vi "Vision Processing (1).vi"(4 "View Processed Image":bool, 5 "Image Size":i32, 6 "Score Limits":T5={"Rect Coverage"=60.0, "X Edge Strength"=40.0, "Y Edge Strength"=60.0, "Center"=75.0, "Outer"=75.0}, 7 "Camera Type":enum16{"206", "1011"}(ring)=enum."1011", 8 "Area Size Limit %":dbl=0.5, 9 "Particle Count Limit":i32=8, 10 "Image Filter Values":T2={"Hue"=89, "Saturation"=255, "Luminance"=255, "Margins"={"Hue"=80, "Val"=0, "Sat"=0}} {"Margins"."Sat" scale=0.0..80.0; "Margins"."Val" scale=0.0..80.0; "Margins"."Hue" scale=0.0..80.0; "Hue" scale=0.0..255.0}, 11 "Image In":T4) -> (1 "Image Filter Ranges":T1, 2 "Processed Image":T4(plugin-control), 3 "Target Info":T6(array[cluster]))   [LabVIEW 2013]
uses:
  <vilib>/vision/Image Controls.llb/IMAQ Image.ctl
  <vilib>/vision/NI_Vision_Development_Module.lvlib
panel:
  in  "Image Filter":T3
  in  "Processing":enum32{"Color", "Monochrome"}(tab)
  in  "Range":cluster{"Lower value":sgl, "Upper value":sgl}={"Lower value"=150.0, "Upper value"=255.0} {"Lower value" scale=0.0..255.0; "Upper value" scale=0.0..255.0}
  in  "View":bool
  out "Original Image":T4(plugin-control)
  # "<--- Disabled"
  # "Lower/Upper"
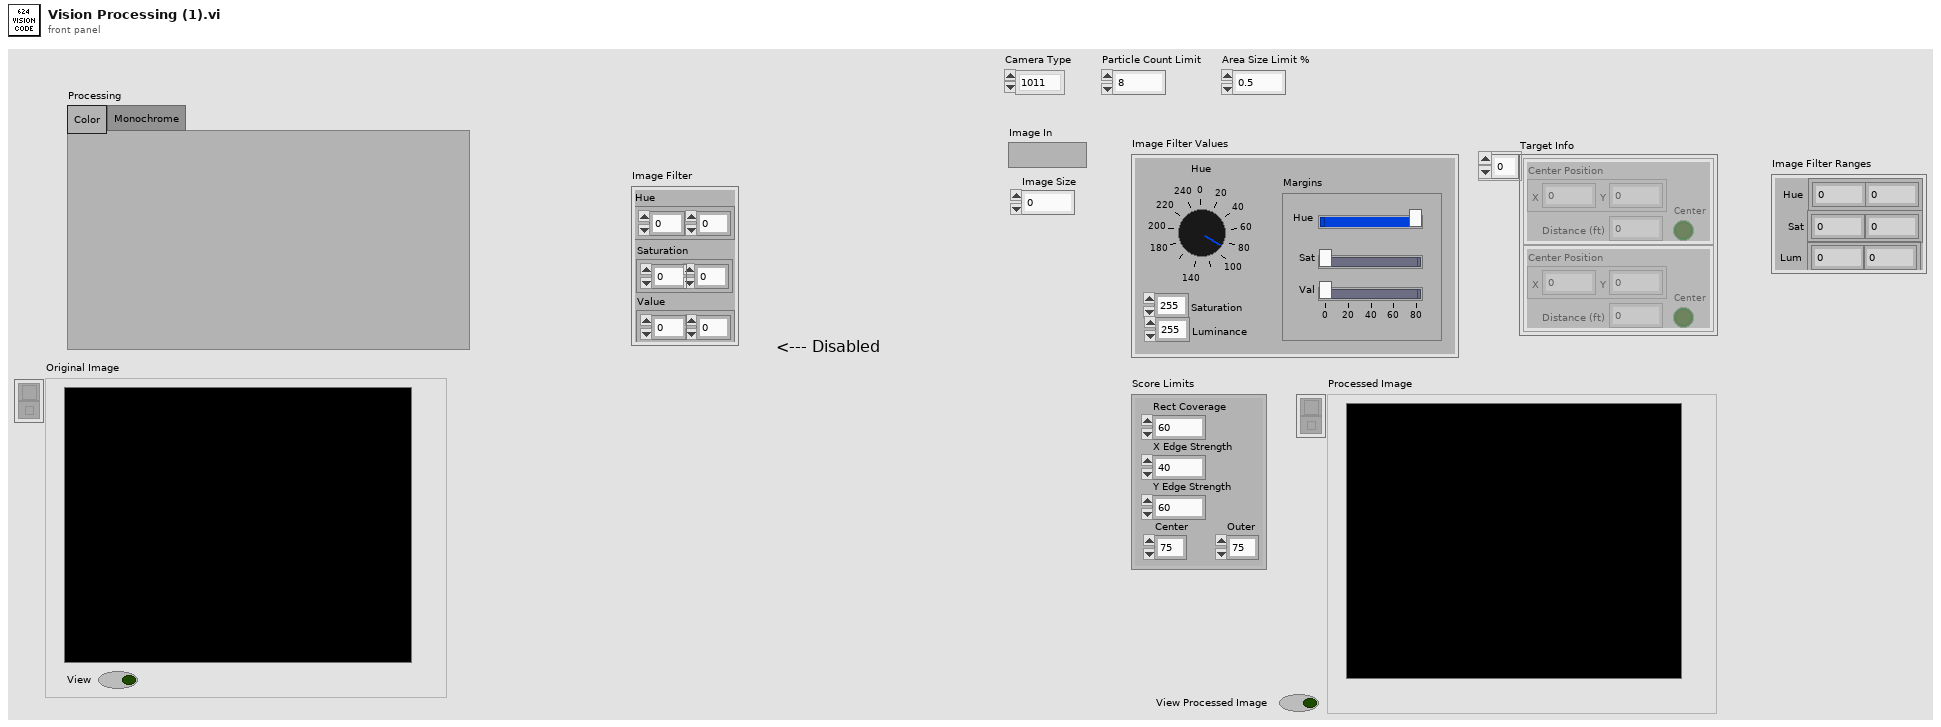
[diagram p1: front panel]
types:
  T1 = cluster{"Hue":cluster{i32, i32}, "Sat":cluster{i32, i32}, "Lum":cluster{i32, i32}}
  T2 = cluster{"Hue":i32, "Saturation":i32, "Luminance":i32, "Margins":cluster{"Hue":i32, "Val":i32, "Sat":i32}}
  T3 = cluster{"Hue":cluster{i32, i32}, "Saturation":cluster{i32, i32}, "Value":cluster{i32, i32}}
  T4 = typedef "IMAQ Image.ctl" = refnum<image>
  T5 = cluster{"Rect Coverage":dbl, "X Edge Strength":dbl, "Y Edge Strength":dbl, "Center":dbl, "Outer":dbl}
  T6 = cluster{"Center Position":cluster{"X":dbl, "Y":dbl}, "Distance (ft)":dbl, "Center":bool}[]
  T7 = cluster{"Position":cluster{"X":dbl, "Y":dbl}, "Distance (ft)":dbl, "Center":bool}[]
  T8 = typedef "Image Type" = u32
  T9 = cluster{cluster{"Left":dbl, "Top":dbl, "Right":dbl, "Bottom":dbl}, "Scores":dbl[], cluster{"Long":dbl, "Short":dbl}}[]
  T10 = cluster{"Target Center (-1 to 1)":cluster{"X":dbl, "Y":dbl}, "Distance (ft)":dbl, "Center Target":bool}
  T11 = cluster{"Target Center (-1 to 1)":cluster{"X":dbl, "Y":dbl}, "Distance (ft)":dbl, "Center Target":bool}[]
  T12 = cluster{"Left":dbl, "Top":dbl, "Right":dbl, "Bottom":dbl}
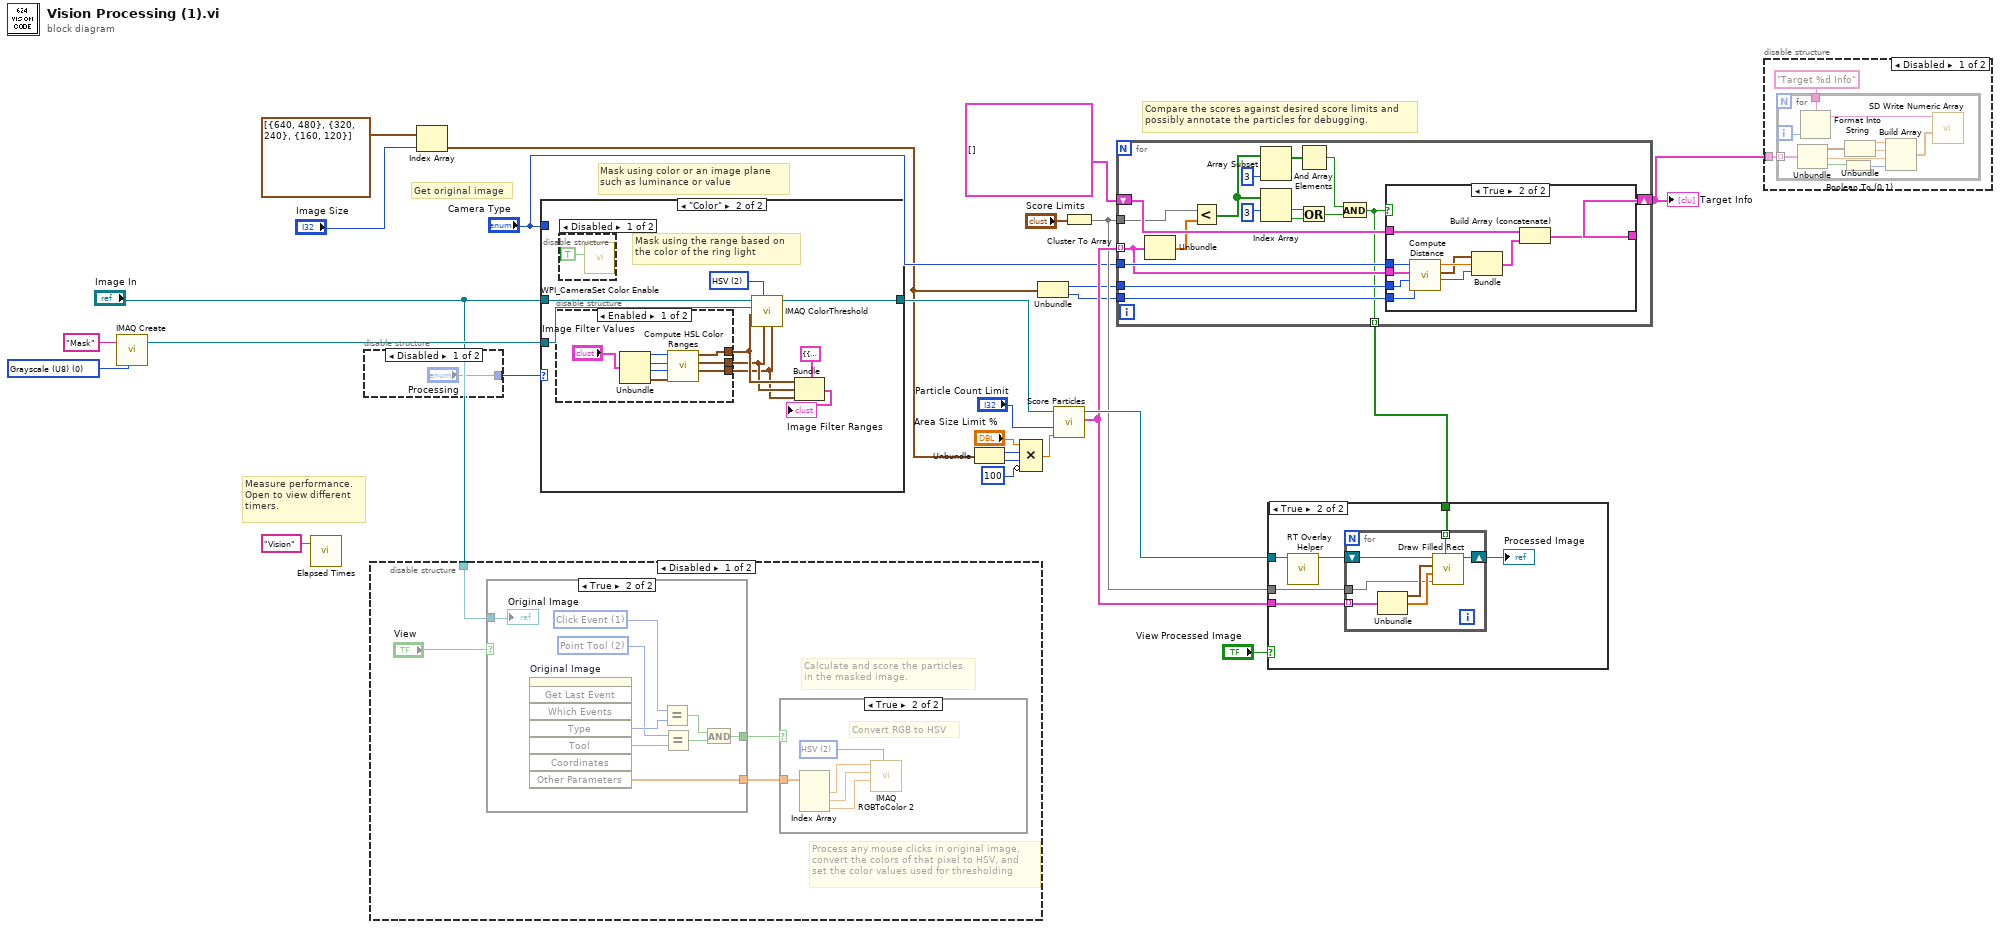
[diagram p0: block diagram]
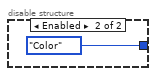
[diagram p8: hidden frame]
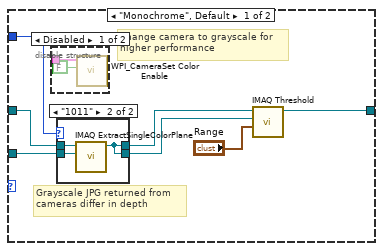
[diagram p9: hidden frame]
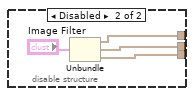
[diagram p12: hidden frame]
diagram:
  w27 = T8 0 items=["Grayscale (U8)", "Grayscale (I16)", "Grayscale (SGL)", "Complex (CSG)", "RGB (U32)", "HSL (U32)", "RGB (U64)", "Grayscale (U16)"] ("Image Type")
  # "Compare the scores against desired score limits and\npossibly annotate the particles for debugging."
  # "Mask using color or an image plane\nsuch as luminance or value"
  # "Get original image"
  # "Measure performance.\nOpen to view different\ntimers."
  n1 = call "IMAQ Create"("Image Name"="Mask", "Image Type"=w27) -> ("New Image"=w25:T4)  [unwired: 2 in, 2 out]
  n2 = call "Elapsed Times.vi"("Call Name"="Vision") -> ()  [unwired: 2 in, 1 out]
  n3 = disable-structure shown="Disabled" {
    disable-tunnel: ["Processing" enum32{"Color", "Monochrome"}."Color" ("Processing 2")] -> w22
    frame Disabled {
    }
    frame Enabled {
    }
  }
  n4 = disable-structure shown="Disabled" {
    disable-tunnel: "Image In" -> [w30 _]
    frame Disabled {
      # "Process any mouse clicks in original image,\nconvert the colors of that pixel to HSV, and\nset the color values used for thresholding"
      # "Calculate and score the particles\nin the masked image."
      n5 = case shown="True" "View" {
        tunnel: w30 -> [_ w47]
        tunnel: [_ w42] -> w32
        tunnel: [_ w39] -> w31
        frame False {
        }
        frame True {
          w40 = 2 items=["None", "Selection Tool", "Point Tool", "Line Tool", "Rectangle Tool", "Oval Tool", "Polygon Tool", "ClosedFreehandTool", "Annulus Tool", "Rotated Rectangle Tool", "Zoom Tool", "Pan Tool", "Polyline Tool", "Freehand Tool"] ("Tool")
          w41 = 1 items=["No Event"=0, "Click Event"=1, "Draw Event"=2, "Size Event"=4, "Scroll Event"=5, "Double Click Event"=8] ("Type")
          n6 = invoke on="Original Image" class="ImageControl" method="Get Last Event"() -> ("Type"=w43:i32, "Tool"=w46:i32, "Other Parameters"=w39:sgl[])  [unwired: 8 in, 5 out]
          n7 = Equal?(x=w41, y=w43) -> (x = y?=w44:bool)
          n8 = Equal?(x=w40, y=w46) -> (x = y?=w45:bool)
          n9 = And(x=w44, y=w45) -> (x .and. y?=w42:bool)
          "Original Image" <- w47
        }
      }
      n10 = case shown="True" w32 {
        tunnel: w31 -> [_ w38]
        frame False {
        }
        frame True {
          w37 = u16 2 items=["RGB", "HSL", "HSV", "HSI", "CIE L*a*b*", "CIE XYZ"] ("Color Mode")
          # "Convert RGB to HSV"
          n11 = Index Array(array=w38) -> (element #1=w36:sgl, element #2=w35:sgl, element #3=w34:sgl)  [unwired: 3 in]
          n12 = call "IMAQ RGBToColor 2"("Color Mode"=w37, "Blue value"=w34, "Green value"=w35, "Red value"=w36) -> ()  [unwired: 4 in, 4 out]
        }
      }
    }
    frame Enabled {
    }
  }
  n13 = Index Array(array=cluster{i32, i32}[] [{640, 480}, {320, 240}, {160, 120}], index="Image Size") -> (element=w15:cluster{i32, i32})
  n14 = case shown="\"Color\"" w22 {
    tunnel: "Image In" -> [w52 w70]
    tunnel: [w53 w69] -> w18
    tunnel: w25 -> [w51 w67]
    tunnel: "Camera Type" -> [w50 _]
    frame "Monochrome", Default {
      # "Grayscale JPG returned from\ncameras differ in depth"
      # "Change camera to grayscale for\nhigher performance"
      n15 = disable-structure shown="Disabled" {
        disable-tunnel: _ -> [w55 _]
        frame Disabled {
          n16 = call <vilib>:"WPI_CameraSet Color Enable.vi"("Color Enabled"=FALSE, "CameraDevRef"=w55) -> ()  [unwired: 8 in, 2 out]
        }
        frame Enabled {
        }
      }
      n17 = case shown="\"1011\"" w50 {
        tunnel: w52 -> [w58 w61]
        tunnel: w51 -> [w57 w60]
        tunnel: [w58 w59] -> w49
        tunnel: [w57 w59] -> w48
        frame "206", Default {
        }
        frame "1011" {
          n18 = call "IMAQ ExtractSingleColorPlane"("Image Dst"=w60, "Image Src"=w61) -> ("Image Dst Out"=w59:T4)  [unwired: 8 in, 1 out]
        }
      }
      n19 = call "IMAQ Threshold"("Range"="Range", "Image Dst"=w48, "Image Src"=w49) -> ("Image Dst Out"=w53:T4)  [unwired: 3 in, 5 out]
    }
    frame "Color" {
      w68 = u16 2 items=["RGB", "HSL", "HSV", "HSI"] ("Color Mode")
      # "Mask using the range based on\nthe color of the ring light"
      n20 = disable-structure shown="Enabled" {
        disable-tunnel: [w78 w80] -> w63
        disable-tunnel: [w77 w79] -> w62
        disable-tunnel: [w76 w81] -> w64
        frame Enabled {
          n21 = Unbundle("Image Filter Values") -> ("Hue"=w74:i32, "Saturation"=w73:i32, "Luminance"=w72:i32, "Margins"=w71:cluster{"Hue":i32, "Val":i32, "Sat":i32})
          n22 = call "Compute HSL Color Ranges.vi"("Margins"=w71, "Luminance"=w72, "Saturation"=w73, "Hue"=w74) -> ("Lum Range"=w77:cluster{i32, i32}, "Sat Range"=w78:cluster{i32, i32}, "Hue Range"=w76:cluster{i32, i32})  [unwired: 5 in]
        }
        frame Disabled {
          n23 = Unbundle("Image Filter") -> ("Hue"=w81:cluster{i32, i32}, "Saturation"=w80:cluster{i32, i32}, "Value"=w79:cluster{i32, i32})
        }
      }
      n24 = disable-structure shown="Disabled" {
        frame Disabled {
          n25 = call <vilib>:"WPI_CameraSet Color Enable.vi"("Color Enabled"=TRUE) -> ()  [unwired: 9 in, 2 out]
        }
        frame Enabled {
        }
      }
      n26 = call "IMAQ ColorThreshold"("Blue or Luma or Val or Inten Range"=w62, "Green or Sat Range"=w63, "Color Mode"=w68, "Red or Hue Range"=w64, "Image Dst"=w67, "Image Src"=w70) -> ("Image Dst Out"=w69:T4)  [unwired: 4 in, 1 out]
      n27 = Bundle(cluster=T1 {"Hue"={0, 0}, "Sat"={0, 0}, "Lum"={0, 0}} ("Image Filter Ranges"), "Hue"=w64, "Sat"=w63, "Lum"=w62) -> (→"Image Filter Ranges":T1)
    }
  }
  n28 = Unbundle(w15) -> (w9:i32, w8:i32)
  n29 = Compound Arithmetic op=MULTIPLY("Area Size Limit %", w9, w8, invert 100 ("length")) -> (w6:dbl)
  n30 = Unbundle(w15) -> (w4:i32, w3:i32)
  n31 = call "Score Particles.vi"("Area Size Limit"=w6, "Particle Count Limit"="Particle Count Limit", "Image Refnum in"=w18) -> ("Scored Particle Info"=w20:T9, "Image Refnum out"=w21:T4)  [unwired: 7 in]
  n32 = Cluster To Array(cluster="Score Limits") -> (array=w19:dbl[])
  n33 = for {
    shift-right: [w99] -> w1
    shift-left: T7 [] -> [w100]
    tunnel: w4 -> [w98]
    tunnel: w20 -> [w93] mode=indexing
    tunnel: w19 -> [w95]
    tunnel: "Camera Type" -> [w97]
    tunnel: w3 -> [w94]
    tunnel: [w84] -> w16 mode=indexing
    n34 = Unbundle(w93) -> ("Scores"=w96:dbl[])  [unwired: 2 out]
    n35 = Less?(x=w95, y=w96) -> (x < y?=w85:bool[])
    n36 = Array Subset(array=w85, length=3) -> (w87:bool[])  [unwired: 1 in]
    n37 = Index Array(array=w85, index #1=3 ("length")) -> (element #1=w89:bool, element #2=w90:bool)  [unwired: 1 in]
    n38 = And Array Elements(Boolean array=w87) -> (logical AND=w92:bool)
    n39 = Or(x=w89, y=w90) -> (x .or. y?=w91:bool)
    n40 = And(x=w92, y=w91) -> (x .and. y?=w84:bool)
    n41 = case shown="True" w84 {
      tunnel: w100 -> [w101 w111]
      tunnel: [w101 w110] -> w99
      tunnel: w98 -> [_ w108]
      tunnel: w97 -> [_ w106]
      tunnel: w94 -> [_ w105]
      tunnel: w93 -> [_ w103]
      frame False {
      }
      frame True {
        n42 = call "Compute Distance.vi"("Y Image Resolution"=w105, "X Image Resolution"=w108, "Particle Scores"=w103, "Camera Type"=w106) -> ("Center Target"=w102:bool, "Target Center (-1 to 1)"=w104:cluster{"X":dbl, "Y":dbl}, "Distance (ft)"=w107:dbl)  [unwired: 5 in]
        n43 = Bundle("Target Center (-1 to 1)"=w104, "Distance (ft)"=w107, "Center Target"=w102) -> (w109:T10)  [unwired: 1 in]
        n44 = Build Array (concatenate)(w111, w109) -> (w110:T11)
      }
    }
  }
  "Target Info" <- w1
  n45 = case shown="True" "View Processed Image" {
    tunnel: w21 -> [_ w114]
    tunnel: w20 -> [_ w116]
    tunnel: w19 -> [_ w115]
    tunnel: w16 -> [_ w112]
    frame False {
    }
    frame True {
      n46 = call "RT Overlay Helper.vi"("Refnum in"=w114) -> ("Refnum out"=w117:T4)  [unwired: 10 in]
      n47 = for {
        shift-right: [w123] -> w113
        shift-left: w117 -> [w124]
        tunnel: w116 -> [w120] mode=indexing
        tunnel: w115 -> [w119]
        tunnel: w112 -> [w118] mode=indexing
        n48 = Unbundle(w120) -> (w121:T12, "Scores"=w122:dbl[])  [unwired: 1 out]
        n49 = call "Draw Filled Rect.vi"("Limit Passed"=w118, "Limits"=w119, "Scores"=w122, "Bounding Box"=w121, "image in"=w124) -> ("image out"=w123:T4)  [unwired: 6 in]
      }
      "Processed Image" <- w113
    }
  }
  n50 = disable-structure shown="Disabled" {
    disable-tunnel: w1 -> [w125 _]
    frame Disabled {
      n51 = for {
        tunnel: w125 -> [w137] mode=indexing
        tunnel: "Target %d Info" ("Name") -> [w136]
        i -> [w133]
        n52 = Unbundle(w137) -> ("Position"=w134:cluster{"X":dbl, "Y":dbl}, "Distance (ft)"=w129:dbl, "Center"=w132:bool)
        n53 = Format Into String(format string=w136, w133) -> (resulting string=w135:string)  [unwired: 2 in, 1 out]
        n54 = Boolean To (0,1)(Boolean=w132) -> (0, 1=w128:i16)
        n55 = Unbundle(w134) -> ("X"=w131:dbl, "Y"=w130:dbl)
        n56 = Build Array(w131, w130, w129, w128) -> (w127:dbl[])
        n57 = call <vilib>:"SD Write Numeric Array.vi"("Numeric Array"=w127, "Name"=w135) -> ()  [unwired: 8 in, 2 out]
      }
    }
    frame Enabled {
    }
  }
